vi "UI.Sequence.GetRowWidths.vi"(8 "error in (no error)":errorcluster, 10 "Numeric":u32, 11 "MulticolumnListbox in":refnum<vi>) -> (0 "error out":errorcluster, 2 "Array":T1[](array[typedef]), 3 "MulticolumnListbox out":refnum<vi>)   [LabVIEW 2013]
uses:
  <vilib>/Utility/miscctls.llb/LVBoundsTypeDef.ctl
  <vilib>/Utility/miscctls.llb/LVRowAndColumnTypeDef.ctl
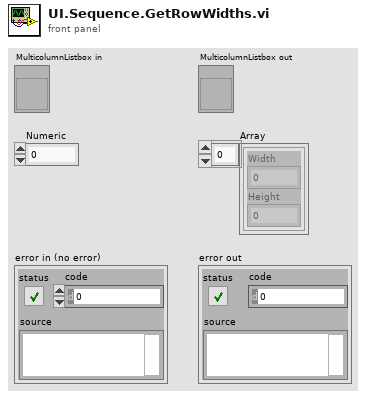
[diagram p1: front panel]
types:
  T1 = typedef "LVBoundsTypeDef.ctl" = cluster{"Width":u32, "Height":u32}
  T2 = typedef "LVRowAndColumnTypeDef.ctl" = cluster{"Row":i32, "Column":i32}
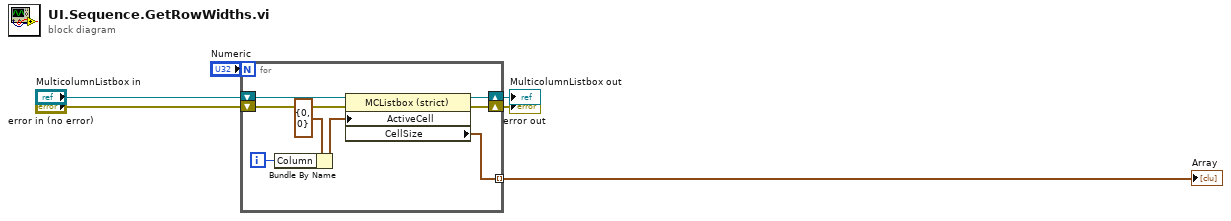
[diagram p0: block diagram]
diagram:
  n1 = for {
    N: "Numeric" -> [_]
    shift-right: [w11] -> w4
    shift-left: "MulticolumnListbox in" -> [w12]
    shift-right: [w13] -> w2
    shift-left: "error in (no error)" -> [w14]
    tunnel: [w7] -> w6 mode=indexing
    i -> [w10]
    n2 = Bundle By Name(cluster=T2 {"Row"=0, "Column"=0} ("Active Cell:Active Cell"), "Column"=w10) -> (w8:T2)
    n3 = property class="MCListbox (strict)"(reference=w12, error in=w14, "ActiveCell"=w8) -> (reference out=w11:refnum<vi>, error out=w13:errorcluster, "CellSize"=w7:T1)
  }
  "Array" <- w6
  "MulticolumnListbox out" <- w4
  "error out" <- w2
